vi "HandShaking.vi"(6 "Elapsed Time":u32, 8 "error in (no error)":errorcluster, 10 "Event Sources":T1, 11 "PostUUT in":refnum<class "PostUUT.lvclass">) -> (0 "error out":errorcluster, 3 "PostUUT out":refnum<class "PostUUT.lvclass">)   [LabVIEW 2021, in "OPC UA.lvlib" / "PostUUT.lvclass"]
uses:
  PostUUT.lvclass
  PostUUT.lvclass/PostUUT.ctl
  <vilib>/addons/TestStand/_TSUtility.llb/TestStand - Get Property Value (String).vi
  OPC UA/OPC UA.lvclass
  d29dd8da-47f8-4898-8208-0e3379922ad0.vi
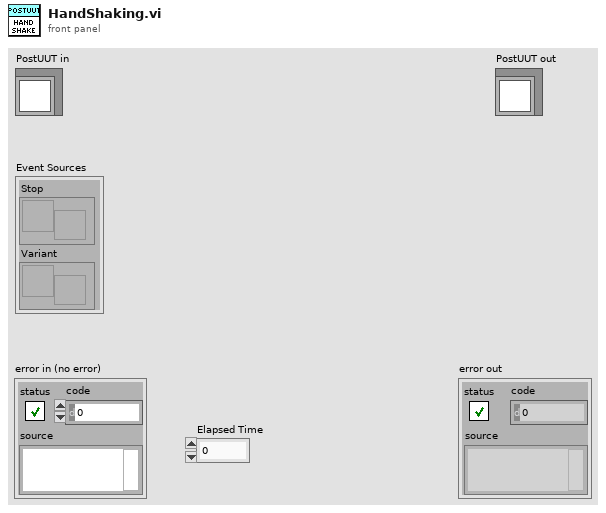
[diagram p1: front panel]
types:
  T1 = cluster{"Stop":refnum<user-event>, "Variant":refnum<user-event>}
  T2 = typedef "PostUUT.lvclass/Rx PostUUT.ctl" = cluster{"ResultsAck":bool, "Reset":bool, "Stop":bool, "FaultCode":u32}
  T3 = typedef "OPC UA.lvlib/PostUUT.lvclass/Tx PostUUT.ctl" = cluster{"ResultsReady":bool, "Results":u32, "ElapsedTime":i32, "TimeCompleted":i32[], "Fault":bool, "Timeout":bool, "Heartbeat":bool}
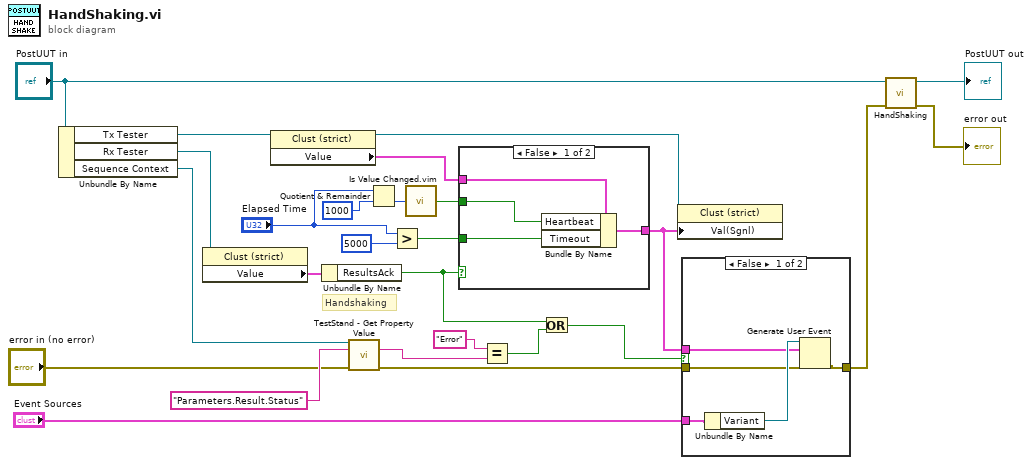
[diagram p0: block diagram]
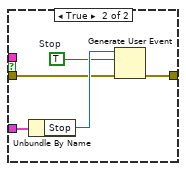
[diagram p2: hidden frame]
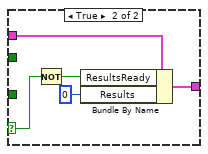
[diagram p3: hidden frame]
diagram:
  # "Handshaking"
  n1 = Unbundle By Name("PostUUT in") -> ("Tx Tester"=w21:refnum<vi>, "Rx Tester"=w22:refnum<vi>, "Sequence Context"=w10:refnum<k7>)
  n2 = property class="Clust (strict)"(reference=w22) -> ("Value"=w23:T2)  [unwired: 1 in, 2 out]
  n3 = property class="Clust (strict)"(reference=w21) -> (reference out=w24:refnum<vi>, "Value"=w25:T3)  [unwired: 1 in, 1 out]
  n4 = Unbundle By Name(w23) -> ("ResultsAck"=w9:bool)
  n5 = call-poly <vilib>:"TestStand - Get Property Value.vi"("Sequence Context In"=w10, "Lookup String"="Parameters.Result.Status", "error in (no error)"="error in (no error)") -> ("Value"=w6:string, "error out"=w11:errorcluster)  [unwired: 10 in, 1 out]
  n6 = Quotient & Remainder(x="Elapsed Time", y=u32 1000) -> (floor(x/y)=w3:u32)  [unwired: 1 out]
  n7 = Greater?(x="Elapsed Time", y=u32 5000) -> (0:w18:bool)
  n8 = call "Is Value Changed.vim"("value"=w3) -> ("changed or first call?"=w1:bool)
  n9 = case shown="False" w9 {
    selector: w9 -> [_ w32]
    tunnel: w25 -> [w30 w34]
    tunnel: [w29 w33] -> w15
    tunnel: w18 -> [w28 _]
    tunnel: w1 -> [w27 _]
    frame False {
      n10 = Bundle By Name(cluster=w30, "Heartbeat"=w27, "Timeout"=w28) -> (w29:T3)
    }
    frame True {
      n11 = Not(x=w32) -> (.not. x?=w31:bool)
      n12 = Bundle By Name(cluster=w34, "ResultsReady"=w31, "Results"=0) -> (w33:T3)
    }
  }
  n13 = Equal?(x="Error" ("Lookup String"), y=w6) -> (x = y?=w7:bool)
  n14 = Or(x=w9, y=w7) -> (x .or. y?=w8:bool)
  n15 = property class="Clust (strict)"(reference=w24, "Val(Sgnl)"=w15) -> ()  [unwired: 1 in, 2 out]
  n16 = case shown="False" w8 {
    tunnel: "Event Sources" -> [w40 w45]
    tunnel: w15 -> [w38 _]
    tunnel: w11 -> [w37 w42]
    tunnel: [w36 w41] -> w14
    frame False {
      n17 = Unbundle By Name(w40) -> ("Variant"=w39:refnum<user-event>)
      n18 = Generate User Event(user event=w39, event data cluster=w38, error in=w37) -> (error out=w36:errorcluster)  [unwired: 1 in, 1 out]
    }
    frame True {
      w43 = TRUE  # Stop
      n19 = Unbundle By Name(w45) -> ("Stop"=w44:refnum<user-event>)
      n20 = Generate User Event(user event=w44, event data cluster=w43, error in=w42) -> (error out=w41:errorcluster)  [unwired: 1 in, 1 out]
    }
  }
  n21 = call-parent "HandShaking.vi"("error in (no error)"=w14, "OPC UA in"="PostUUT in") -> ("error out"=→"error out":errorcluster, "OPC UA out"=→"PostUUT out":refnum<class "PostUUT.lvclass">)  [unwired: 8 in]
